vi "ConfigFromToFile.vi"(8 "error in":errorcluster, 9 "Configuration File Path":path, 10 "ReadFromFile?":bool, 11 "Default Values":cluster{"Comport":string, "Baud Rate":u32}={"Comport"="COM4", "Baud Rate"=57600}) -> (0 "error out":errorcluster={"status"=TRUE, "code"=-1073807339, "source"="VISA Read in FirmataClient.lvlib:Initialize.vi"}, 3 "Config Out":cluster{"Comport":string, "Baud Rate":u32}={"Comport"="COM4", "Baud Rate"=57600})   [LabVIEW 2020, in "FirmataClient.lvlib"]
doc: "Read or Write Firmata Client Serial Communication configuration from / to a file (e.g. comport, baud rate, ...)"
uses:
  FirmataClient.lvlib
  <vilib>/Utility/config.llb/Read Key (String).vi
  <vilib>/Utility/config.llb/Write Key (String).vi
  <vilib>/Utility/config.llb/NI_LVConfig.lvlib
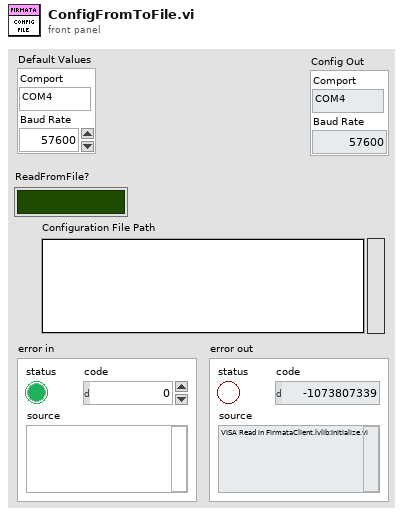
[diagram p1: front panel]
types:
  T1 = typedef "NI_LVConfig.lvlib/Config Data RefNum.ctl" = refnum<k1>
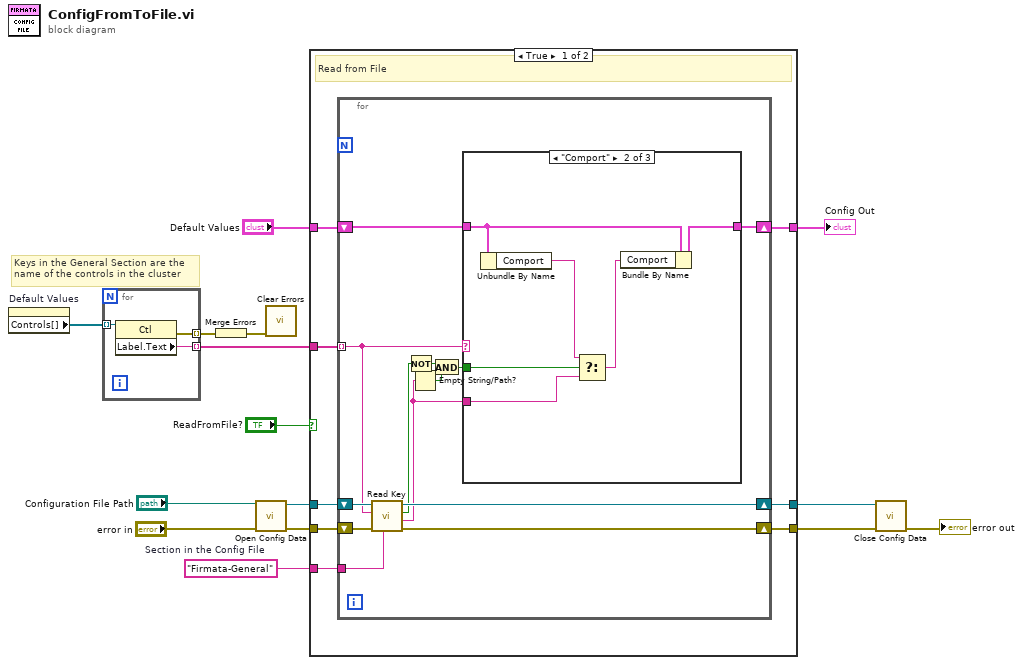
[diagram p0: block diagram]
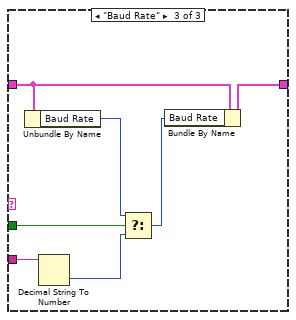
[diagram p3: hidden frame]
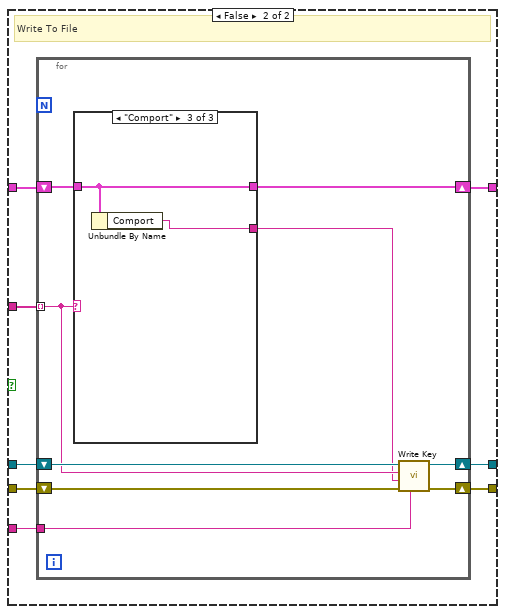
[diagram p4: hidden frame]
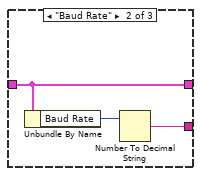
[diagram p6: hidden frame]
diagram:
  w13 = "Firmata-General"  # Section in the Config File
  # "Keys in the General Section are the \nname of the controls in the cluster"
  n1 = property on="Default Values" class="Clust (strict)"() -> ("Controls[]"=w5:refnum<vi>[])  [unwired: 2 in, 2 out]
  n2 = for {
    tunnel: w5 -> [w18] mode=indexing
    tunnel: [w17] -> w4 mode=indexing
    tunnel: [w16] -> w2 mode=indexing
    n3 = property class="Ctl"(reference=w18) -> (error out=w16:errorcluster, "Label.Text"=w17:string)  [unwired: 1 in, 1 out]
  }
  n4 = Merge Errors(w2) -> (w1:errorcluster)
  n5 = call <vilib>:"Open Config Data.vi"("error in (no error)"="error in", "configuration file path"="Configuration File Path") -> ("error out"=w15:errorcluster, "refnum"=w14:T1)  [unwired: 7 in, 1 out]
  n6 = call <vilib>:"Clear Errors.vi"("error in (no error)"=w1) -> ()  [unwired: 5 in, 2 out]
  n7 = case shown="True" "ReadFromFile?" {
    tunnel: w15 -> [w26 w61]
    tunnel: w14 -> [w25 w60]
    tunnel: w4 -> [w24 w59]
    tunnel: w13 -> [w23 w58]
    tunnel: [w22 w57] -> w12
    tunnel: [w21 w56] -> w11
    tunnel: "Default Values" -> [w20 w55]
    tunnel: [w19 w54] -> w3
    frame True {
      # "Read from File"
      n8 = for {
        shift-right: [w36] -> w22
        shift-left: w26 -> [w39]
        tunnel: w24 -> [w37] mode=indexing
        tunnel: w23 -> [w35]
        shift-right: [w34] -> w21
        shift-left: w25 -> [w38]
        shift-right: [w29] -> w19
        shift-left: w20 -> [w28]
        n9 = call-poly <vilib>:"Read Key.vi"("section"=w35, "error in (no error)"=w39, "key"=w37, "refnum"=w38) -> ("error out"=w36:errorcluster, "value"=w27:string, "found?"=w30:bool, "refnum out"=w34:T1)  [unwired: 4 in]
        n10 = Not(x=w30) -> (.not. x?=w32:bool)
        n11 = Empty String/Path?(string/path=w27) -> (empty?=w33:bool)
        n12 = And(x=w32, y=w33) -> (x .and. y?=w31:bool)
        n13 = case shown="\"Comport\"" w37 {
          tunnel: w31 -> [_ w44 w51]
          tunnel: [w40 w45 w52] -> w29
          tunnel: w28 -> [w40 w46 w53]
          tunnel: w27 -> [_ w43 w48]
          frame Default {
          }
          frame "Comport" {
            n14 = Unbundle By Name(w46) -> ("Comport"=w42:string)
            n15 = Select(t=w42, s=w44, f=w43) -> (s? t:f=w41:string)
            n16 = Bundle By Name(cluster=w46, "Comport"=w41) -> (w45:cluster{"Comport":string, "Baud Rate":u32})
          }
          frame "Baud Rate" {
            n17 = Unbundle By Name(w53) -> ("Baud Rate"=w50:u32)
            n18 = Decimal String To Number(string=w48) -> (number=w47:i32)  [unwired: 2 in, 1 out]
            n19 = Select(t=w50, s=w51, f=w47) -> (s? t:f=w49:u32)
            n20 = Bundle By Name(cluster=w53, "Baud Rate"=w49) -> (w52:cluster{"Comport":string, "Baud Rate":u32})
          }
        }
      }
    }
    frame False {
      # "Write To File"
      n21 = for {
        shift-right: [w67] -> w57
        shift-left: w61 -> [w70]
        tunnel: w59 -> [w68] mode=indexing
        tunnel: w58 -> [w66]
        shift-right: [w65] -> w56
        shift-left: w60 -> [w69]
        shift-right: [w64] -> w54
        shift-left: w55 -> [w63]
        n22 = case shown="\"Comport\"" w68 {
          tunnel: [w71 w74 w76] -> w64
          tunnel: w63 -> [w71 w74 w76]
          tunnel: [_ w73 w75] -> w62
          frame Default {
          }
          frame "Baud Rate" {
            n23 = Unbundle By Name(w74) -> ("Baud Rate"=w72:u32)
            n24 = Number To Decimal String(number=w72) -> (decimal integer string=w73:string)  [unwired: 1 in]
          }
          frame "Comport" {
            n25 = Unbundle By Name(w76) -> ("Comport"=w75:string)
          }
        }
        n26 = call-poly <vilib>:"Write Key.vi"("section"=w66, "error in (no error)"=w70, "value"=w62, "key"=w68, "refnum"=w69) -> ("error out"=w67:errorcluster, "refnum out"=w65:T1)  [unwired: 4 in, 1 out]
      }
    }
  }
  "Config Out" <- w3
  n27 = call <vilib>:"Close Config Data.vi"("error in (no error)"=w12, "refnum"=w11) -> ("error out"=→"error out":errorcluster)  [unwired: 8 in, 1 out]
